vi "ReferenceSyncPoint.vi"(8 "error in":errorcluster) -> (0 "error out":errorcluster, 3 "SynchPointRef":refnum<vi>)   [LabVIEW 2016]
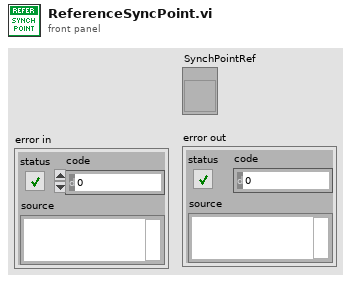
[diagram p1: front panel]
types:
  T1 = enum32{"Invalid", "Standard", "Closed", "Hidden", "Minimized", "Maximized"}
  T2 = enum32{"Bad", "Idle", "Run top level", "Running"}
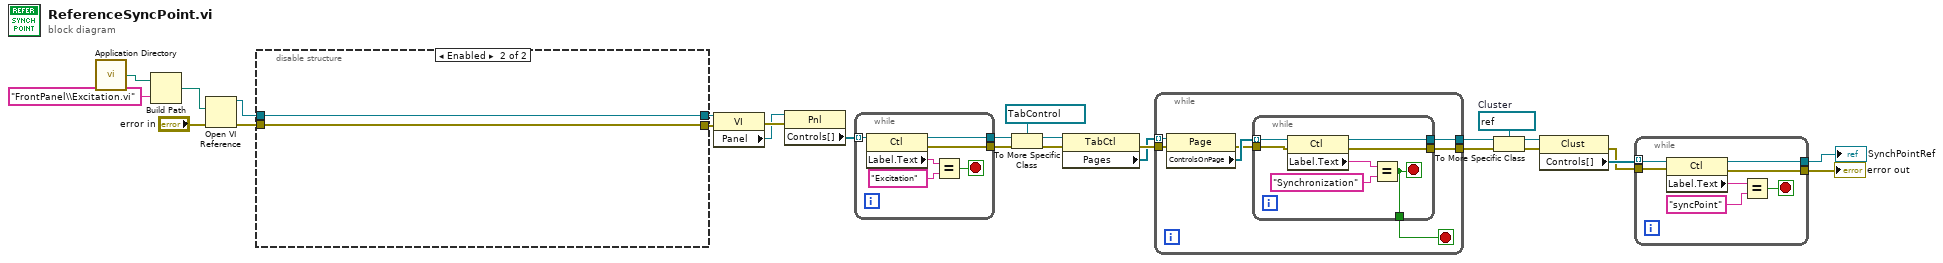
[diagram p0: block diagram]
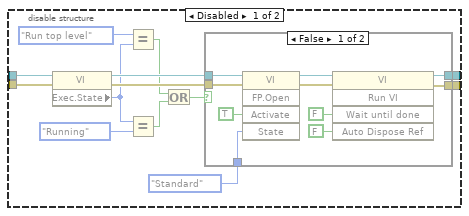
[diagram p2: hidden frame]
diagram:
  w8 = refnum<vi> refnum  # Cluster
  n1 = call <vilib>:"Application Directory.vi"() -> ("Application Directory"=w25:path)
  n2 = Build Path(base path=w25, name or relative path="FrontPanel\\Excitation.vi") -> (appended path=w24:path)
  n3 = Open VI Reference(vi path=w24, error in (no error)="error in") -> (vi reference=w20:refnum<vi>, error out=w19:errorcluster)  [unwired: 4 in]
  n4 = disable-structure shown="Enabled" {
    disable-tunnel: [w40 w53] -> w22
    disable-tunnel: [w39 w54] -> w21
    disable-tunnel: w20 -> [w38 w54]
    disable-tunnel: w19 -> [w36 w53]
    frame Disabled {
      n5 = property class="VI"(reference=w38, error in=w36) -> (reference out=w37:refnum<vi>, error out=w35:errorcluster, "Exec.State"=w30:T2)
      n6 = Equal?(x=T2."Run top level" ("Execution:State"), y=w30) -> (x = y?=w32:bool)
      n7 = Equal?(x=w30, y=T2."Running" ("Execution:State")) -> (x = y?=w31:bool)
      n8 = Or(x=w32, y=w31) -> (x .or. y?=w29:bool)
      n9 = case shown="False" w29 {
        tunnel: [w45 w51] -> w40
        tunnel: [w44 w52] -> w39
        tunnel: w37 -> [w43 w52]
        tunnel: w35 -> [w42 w51]
        tunnel: T1."Standard" ("State") -> [w41 _]
        frame False {
          n10 = invoke class="VI" method="FP.Open"(reference=w43, error in=w42, "Activate"=TRUE ("Activate?"), "State"=w41) -> (reference out=w47:refnum<vi>, error out=w46:errorcluster)  [unwired: 1 in, 3 out]
          n11 = invoke class="VI" method="Run VI"(reference=w47, error in=w46, "Wait until done"=FALSE ("Wait Until Done"), "Auto Dispose Ref"=FALSE ("Auto Dispose Reference")) -> (reference out=w44:refnum<vi>, error out=w45:errorcluster)  [unwired: 1 in, 3 out]
        }
        frame True {
        }
      }
    }
    frame Enabled {
    }
  }
  n12 = property class="VI"(reference=w21, error in=w22) -> (error out=w27:errorcluster, "Panel"=w12:refnum<vi>)  [unwired: 1 out]
  n13 = property class="Pnl"(reference=w12, error in=w27) -> ("Controls[]"=w18:refnum<vi>[])  [unwired: 2 out]
  n14 = while {
    tunnel: w18 -> [w60] mode=indexing
    tunnel: [w59] -> w11
    tunnel: [w55] -> w10
    stop <- w56 stop-if-true
    n15 = property class="Ctl"(reference=w60) -> (reference out=w59:refnum<vi>, error out=w55:errorcluster, "Label.Text"=w58:string)  [unwired: 1 in]
    n16 = Equal?(x=w58, y="Excitation" ("Label.Text")) -> (x = y?=w56:bool)
  }
  n17 = To More Specific Class(target class=refnum<vi> refnum ("Menus"), reference=w11, error in=w10) -> (specific class reference=w14:refnum<vi>, error out=w17:errorcluster)
  n18 = property class="TabCtl"(reference=w14, error in=w17) -> (error out=w16:errorcluster, "Pages"=w15:refnum<vi>[])  [unwired: 1 out]
  n19 = while {
    tunnel: w15 -> [w67] mode=indexing
    tunnel: [w65] -> w2
    tunnel: [w64] -> w1
    tunnel: w16 -> [w62]
    stop <- w61 stop-if-true
    n20 = property class="Page"(reference=w67, error in=w62) -> (error out=w63:errorcluster, "ControlsOnPage"=w66:refnum<vi>[])  [unwired: 1 out]
    n21 = while {
      tunnel: w66 -> [w74] mode=indexing
      tunnel: [w73] -> w65
      tunnel: [w72] -> w64
      tunnel: w63 -> [w71]
      tunnel: [w68] -> w61
      stop <- w68 stop-if-true
      n22 = property class="Ctl"(reference=w74, error in=w71) -> (reference out=w73:refnum<vi>, error out=w72:errorcluster, "Label.Text"=w70:string)
      n23 = Equal?(x=w70, y="Synchronization" ("Label.Text")) -> (x = y?=w68:bool)
    }
  }
  n24 = To More Specific Class(target class=w8, reference=w2, error in=w1) -> (specific class reference=w7:refnum<vi>, error out=w6:errorcluster)
  n25 = property class="Clust"(reference=w7, error in=w6) -> (error out=w3:errorcluster, "Controls[]"=w5:refnum<vi>[])  [unwired: 1 out]
  n26 = while {
    tunnel: w5 -> [w81] mode=indexing
    tunnel: [w77] -> w4
    tunnel: w3 -> [w76]
    tunnel: [w75] -> w9
    stop <- w78 stop-if-true
    n27 = property class="Ctl"(reference=w81, error in=w76) -> (reference out=w77:refnum<vi>, error out=w75:errorcluster, "Label.Text"=w80:string)
    n28 = Equal?(x=w80, y="syncPoint") -> (x = y?=w78:bool)
  }
  "SynchPointRef" <- w4
  "error out" <- w9
